vi "testevent.vi"() -> ()   [LabVIEW 2011]
uses:
  kernel32.dll
panel:
  in  "布尔":bool
  out "数值":i32
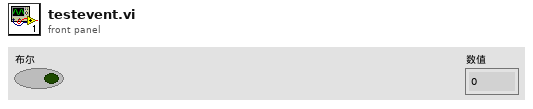
[diagram p1: front panel]
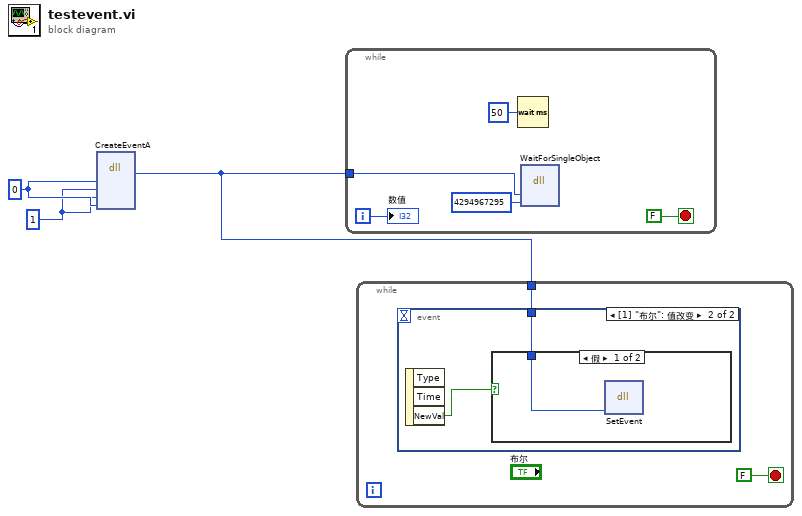
[diagram p0: block diagram]
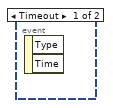
[diagram p2: hidden frame]
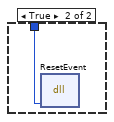
[diagram p3: hidden frame]
diagram:
  w2 = i8 1 ("LPSECURITY_ATTRIBUTES lpEventAttributes")
  w3 = i8 0 ("LPSECURITY_ATTRIBUTES lpEventAttributes")
  n1 = dll-call lib="kernel32.dll" fn="CreateEventA"("LPSECURITY_ATTRIBUTES lpEventAttributes"=w3, "BOOL bManualReset"=w2, "BOOL bInitialState"=w2, "LPCTSTR lpName"=w3) -> ("HANDLE CreateEvent"=w1:i32)  [unwired: 7 in, 2 out]
  n2 = while {
    tunnel: w1 -> [w4]
    i -> [w6]
    stop <- FALSE stop-if-true
    n3 = Wait (ms)(milliseconds to wait=u32 50 ("等待时间（毫秒）")) -> ()  [unwired: 1 out]
    n4 = dll-call lib="kernel32.dll" fn="WaitForSingleObject"("HANDLE hHandle"=w4, "DWORD dwMilliseconds"=u32 4294967295) -> ()  [unwired: 6 in, 2 out]
    "数值" <- w6
  }
  n5 = while {
    tunnel: w1 -> [w9]
    stop <- FALSE stop-if-true
    n6 = event shown="[1] \"布尔\": 值改变" {
      selector: _ -> [_ _]
      dyn-events: _ -> [_ _]
      timeout: _ -> [_ _]
      tunnel: w9 -> [_ w11]
      event Timeout {
        n7 = event-data() -> ()  [unwired: 1 in, 2 out]
      }
      event "布尔": Value Change {
        n8 = event-data() -> ("NewVal"=w12:bool)  [unwired: 1 in, 2 out]
        n9 = case shown="假" w12 {
          tunnel: w11 -> [w13 w14]
          frame False {
            n10 = dll-call lib="kernel32.dll" fn="SetEvent"("参数1"=w13) -> ()  [unwired: 5 in, 2 out]
          }
          frame True {
            n11 = dll-call lib="kernel32.dll" fn="ResetEvent"("参数1"=w14) -> ()  [unwired: 5 in, 2 out]
          }
        }
      }
    }
  }
